vi "Read Loop Async.vi"(11 "VISA GPS in":refnum<class "VISA GPS.lvclass">) -> ()   [LabVIEW 2020, in "VISA GPS.lvlib" / "VISA GPS.lvclass"]
uses:
  VISA GPS.lvclass
  <vilib>/Instr/_visa.llb/VISA Flush IO Buffer Mask.ctl
  VISA GPS.lvclass/VISA GPS.ctl
  nmea/nmea.lvclass
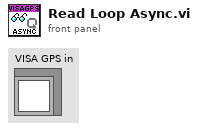
[diagram p1: front panel]
types:
  T1 = typedef "VISA Flush IO Buffer Mask.ctl" = u16
  T2 = typedef "nmea.lvlib/VISA GPS.lvclass/Ref Data.ctl" = cluster{"Close":bool}
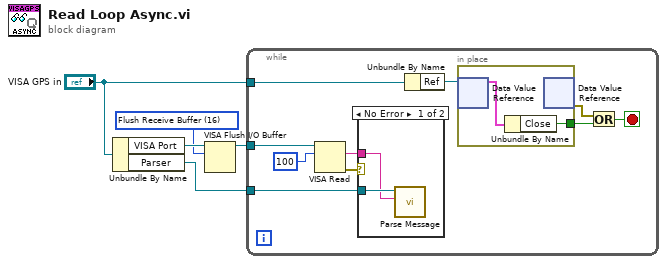
[diagram p0: block diagram]
diagram:
  w1 = T1 16 items=["Flush Receive Buffer"=16, "Write Transmit Buffer to Device"=32, "Flush Receive Buffer (No I/O)"=64, "Flush Transmit Buffer"=128] ("Mask")
  n1 = Unbundle By Name("VISA GPS in") -> ("VISA Port"=w3:refnum<visa-resource-name>, "Parser"=w4:refnum<class "nmea.lvclass">)
  n2 = VISA Flush I/O Buffer(VISA resource name=w3, mask (16)=w1) -> (VISA resource name out=w2:refnum<visa-resource-name>)  [unwired: 1 in, 1 out]
  n3 = while {
    tunnel: "VISA GPS in" -> [w9]
    tunnel: w2 -> [w15]
    tunnel: w4 -> [w13]
    stop <- w7 stop-if-true
    n4 = VISA Read(VISA resource name=w15, byte count=u32 100) -> (read buffer=w11:string, error out=w12:errorcluster)  [unwired: 1 in, 2 out]
    n5 = case shown="No Error" w12 {
      tunnel: w13 -> [w17 _]
      tunnel: w11 -> [w16 _]
      frame No Error {
        n6 = call "Parse Message.vi"("NMEA Message"=w16, "nmea in"=w17) -> ()  [unwired: 8 in, 2 out]
      }
      frame Error {
      }
    }
    n7 = Unbundle By Name(w9) -> ("Ref"=w10:refnum<data-value>)
    n8 = in-place {
      in-place-border: [w18] -> w8
      n9 = in-place-dvr #1(w10) -> (w19:T2)  [unwired: 1 out]
      n10 = Unbundle By Name(w19) -> ("Close"=w18:bool)
      n11 = in-place-dvr #1() -> (w6:errorcluster)  [unwired: 1 in, 1 out]
    }
    n12 = Or(x=w6, y=w8) -> (x .or. y?=w7:bool)
  }
